vi "SUB_TestPoint_Format.vi"(0 "TestPoint_Name":string="TP46", 1 "Lower Limit Voltage":dbl format="%#.6f", 2 "High Limit Voltage":dbl format="%#.6f", 3 "Relay 1 Name":string, 4 "Relay1 H/L":bool=TRUE, 6 "Relay 2 Name":string, 7 "Relay2 H/L":bool=TRUE, 8 "Relay3 Name":string, 9 "Relay3H/L":bool=TRUE, 10 "Measure Ai name":string) -> (14 "output cluster":T1 {"Lower Limit Voltage" format="%#.6f"; "High Limit Voltage" format="%#.6f"})   [LabVIEW 2011]
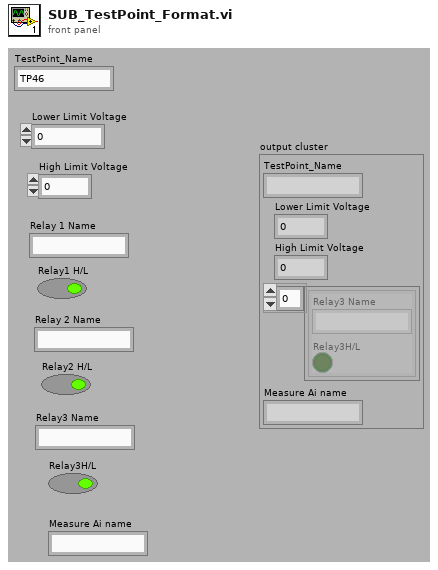
[diagram p1: front panel]
types:
  T1 = cluster{"TestPoint_Name":string, "Lower Limit Voltage":dbl, "High Limit Voltage":dbl, cluster{"Relay3 Name":string, "Relay3H/L":bool}[], "Measure Ai name":string}
  T2 = cluster{"Relay 1 Name":string, "Relay1 H/L":bool}
  T3 = cluster{"Relay 2 Name":string, "Relay2 H/L":bool}
  T4 = cluster{"Relay3 Name":string, "Relay3H/L":bool}[]
  T5 = cluster{"TestPoint_Name":string, "Lower Limit Voltage":dbl, "High Limit Voltage ":dbl, cluster{"Relay3 Name":string, "Relay3H/L":bool}[], "Measure Ai name":string}
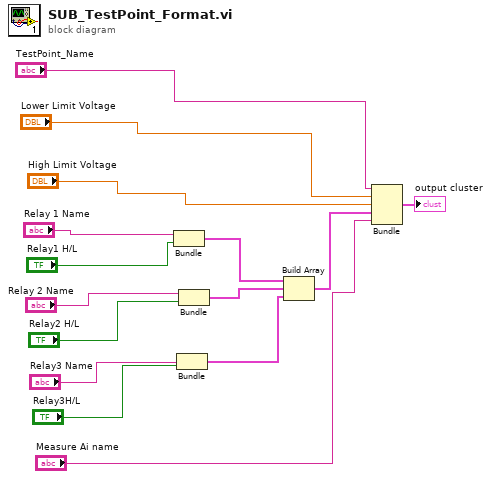
[diagram p0: block diagram]
diagram:
  n1 = Bundle("Relay 1 Name"="Relay 1 Name", "Relay1 H/L"="Relay1 H/L") -> (w9:T2)  [unwired: 1 in]
  n2 = Bundle("Relay3 Name"="Relay3 Name", "Relay3H/L"="Relay3H/L") -> (w7:cluster{"Relay3 Name":string, "Relay3H/L":bool})  [unwired: 1 in]
  n3 = Bundle("Relay 2 Name"="Relay 2 Name", "Relay2 H/L"="Relay2 H/L") -> (w8:T3)  [unwired: 1 in]
  n4 = Build Array(w9, w8, w7) -> (w3:T4)
  n5 = Bundle("TestPoint_Name"="TestPoint_Name", "Lower Limit Voltage"="Lower Limit Voltage", "High Limit Voltage"="High Limit Voltage", w3, "Measure Ai name"="Measure Ai name") -> (→"output cluster":T5)  [unwired: 1 in]
